vi "uTTA_CheckSystemTime.vi"(4 "error in":errorcluster, 7 "VISA in":refnum<visa-resource-name>) -> (0 "error out":errorcluster, 3 "VISA Refnum out":refnum<visa-resource-name>)   [LabVIEW 2021]
panel:
  out "DeltaTime":dbl
  out "uTTA Time":timestamp
  out "Received":string
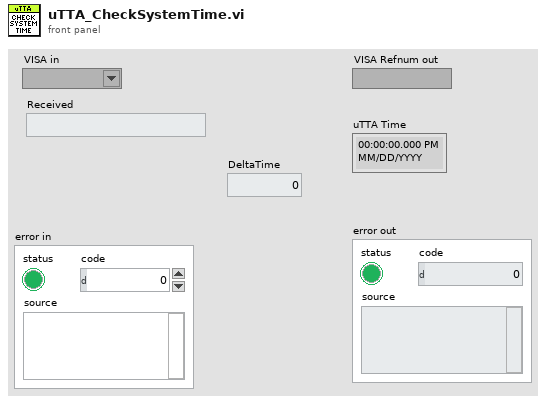
[diagram p1: front panel]
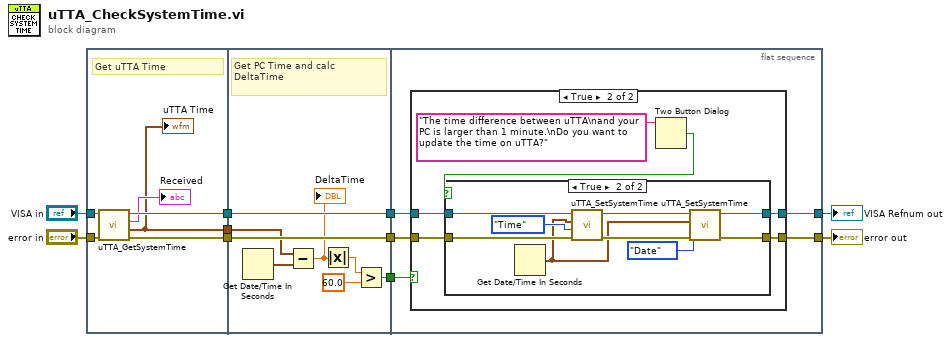
[diagram p0: block diagram]
diagram:
  n1 = flat-sequence {
    tunnel: "VISA in" -> [w16]
    tunnel: "error in" -> [w15]
    tunnel: [w14] -> w10
    tunnel: [w13] -> w9
    tunnel: [w11] -> w8
    tunnel: w10 -> [w24]
    tunnel: w9 -> [w23]
    tunnel: w8 -> [w22]
    tunnel: [w24] -> w7
    tunnel: [w23] -> w6
    tunnel: [w17] -> w5
    tunnel: [w26] -> w2
    tunnel: [w25] -> w1
    tunnel: w7 -> [w27]
    tunnel: w6 -> [w28]
    tunnel: w5 -> [w29]
    frame #0 {
      # "Get uTTA Time"
      n2 = call "uTTA_GetSystemTime.vi"("error in"=w15, "VISA Refnum in"=w16) -> ("error out"=w14:errorcluster, "Timestamp"=w11:timestamp, "Received"=→"Received":string, "VISA Refnum out"=w13:refnum<visa-resource-name>)  [unwired: 2 in]
      "uTTA Time" <- w11
    }
    frame #1 {
      # "Get PC Time and calc DeltaTime"
      n3 = Get Date/Time In Seconds() -> (seconds since 1Jan1904=w21:timestamp)
      n4 = Subtract(x=w22, y=w21) -> (x-y=w18:dbl)
      "DeltaTime" <- w18
      n5 = Absolute Value(x=w18) -> (abs(x)=w20:dbl)
      n6 = Greater?(x=w20, y=60.0) -> (0:w17:bool)
    }
    frame #2 {
      n7 = case shown="True" w29 {
        tunnel: w28 -> [w31 w35]
        tunnel: w27 -> [w30 w34]
        tunnel: [w31 w33] -> w26
        tunnel: [w30 w32] -> w25
        frame False {
        }
        frame True {
          n8 = Two Button Dialog(message="The time difference between uTTA\nand your PC is larger than 1 minute.\nDo you want to update the time on uTTA?") -> (T button?=w36:bool)  [unwired: 2 in]
          n9 = case shown="True" w36 {
            tunnel: w35 -> [w39 w48]
            tunnel: w34 -> [w38 w47]
            tunnel: [w39 w41] -> w33
            tunnel: [w38 w40] -> w32
            frame False {
            }
            frame True {
              n10 = Get Date/Time In Seconds() -> (seconds since 1Jan1904=w43:timestamp)
              n11 = call "uTTA_SetSystemTime.vi"("error in"=w47, "Parameter"=enum16{"Date", "Time", "Date+Time"}."Time", "Time Stamp"=w43, "VISA Refnum in"=w48) -> ("error out"=w44:errorcluster, "VISA Refnum out"=w45:refnum<visa-resource-name>)  [unwired: 6 in]
              n12 = call "uTTA_SetSystemTime.vi"("error in"=w44, "Parameter"=enum16{"Date", "Time", "Date+Time"}."Date", "Time Stamp"=w43, "VISA Refnum in"=w45) -> ("error out"=w40:errorcluster, "VISA Refnum out"=w41:refnum<visa-resource-name>)  [unwired: 6 in]
            }
          }
        }
      }
    }
  }
  "VISA Refnum out" <- w2
  "error out" <- w1
